vi "bundleArregloValores.vi"(8 "error in (no error)":errorcluster, 11 "ValoresControles":string[](array[string])=["marca 1", "modelo 1", "1231321", "", "", "Clase 1", "marca 1", "marca 1", "632131", "marca 1", "modelo 1", "654546"]) -> (0 "error out":errorcluster, 3 "output cluster":T1)   [LabVIEW 2019, in "Sonometro.lvclass"]
uses:
  Sonometro.lvclass
  Base de Datos/BD/Controles/cluster_equipos.ctl
  nombreControlesEquipo.ctl
  Base de Datos/Base de Datos.lvclass
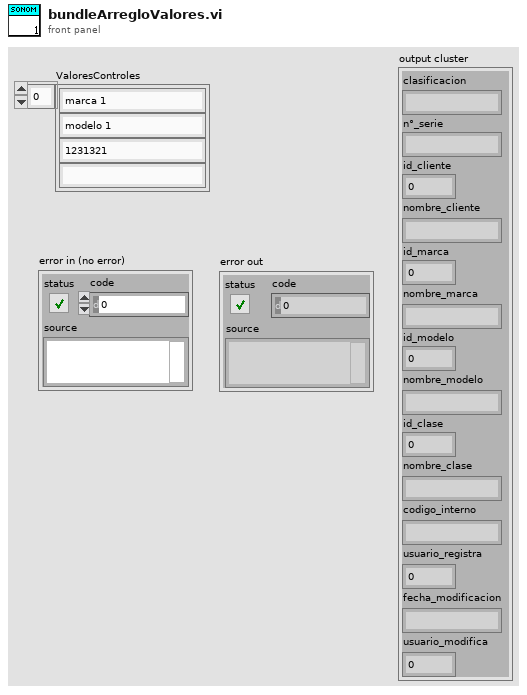
[diagram p1: front panel]
types:
  T1 = typedef "Base de Datos.lvclass/cluster_equipos.ctl" = cluster{"clasificacion":string, "n°_serie":string, "id_cliente":i32, "nombre_cliente":string, "id_marca":i32, "nombre_marca":string, "id_modelo":i32, "nombre_modelo":string, "id_clase":i32, "nombre_clase":string, "codigo_interno":string, "usuario_registra":i32, "fecha_modificacion":string, "usuario_modifica":i32}
  T2 = typedef "Sonometro.lvclass/nombreControlesEquipo.ctl" = string[]
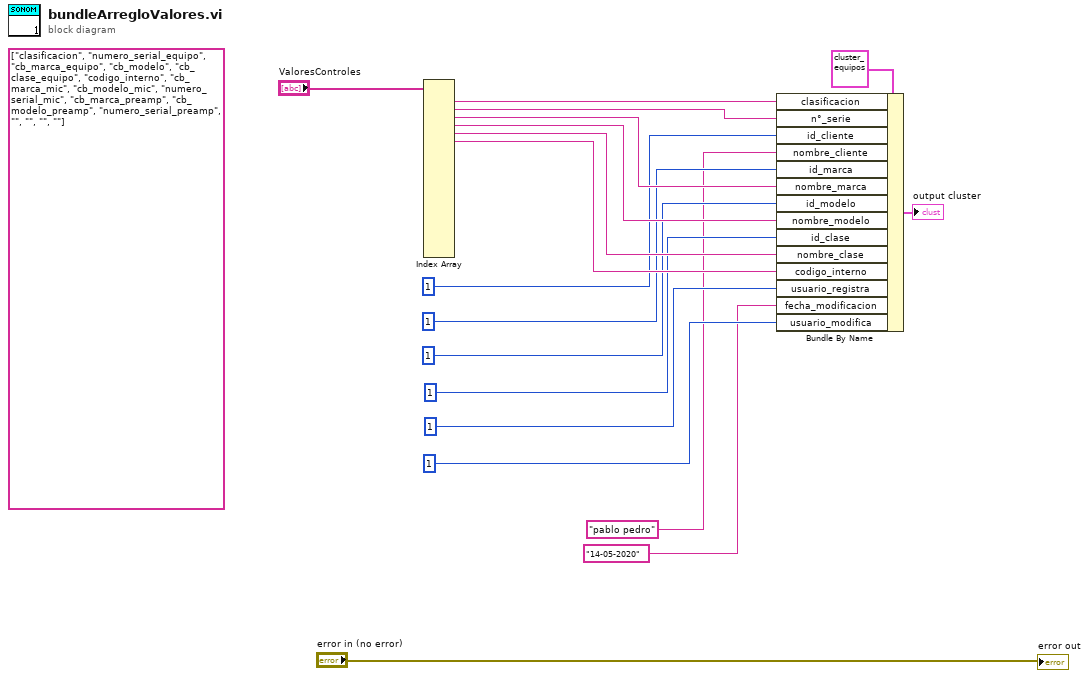
[diagram p0: block diagram]
diagram:
  (unwired) T2 ["clasificacion", "numero_serial_equipo", "cb_marca_equipo", "cb_modelo", "cb_clase_equipo", "codigo_interno", "cb_marca_mic", "cb_modelo_mic", "numero_serial_mic", "cb_marca_preamp", "cb_modelo_preamp", "numero_serial_preamp", "", "", "", ""] ("nombre_controles_equipo")
  n1 = Index Array(array="ValoresControles") -> (element #1=w16:string, element #2=w15:string, element #3=w14:string, element #4=w13:string, element #5=w12:string, element #6=w11:string)  [unwired: 20 in, 14 out]
  n2 = Bundle By Name(cluster=T1 {"clasificacion"="", "n°_serie"="", "id_cliente"=0, "nombre_cliente"="", "id_marca"=0, "nombre_marca"="", "id_modelo"=0, "nombre_modelo"="", "id_clase"=0, "nombre_clase"="", "codigo_interno"="", "usuario_registra"=0, "fecha_modificacion"="", "usuario_modifica"=0} ("cluster_equipos"), "clasificacion"=w16, "n°_serie"=w15, "id_cliente"=1, "nombre_cliente"="pablo pedro", "id_marca"=1 ("id_cliente"), "nombre_marca"=w14, "id_modelo"=1 ("id_cliente"), "nombre_modelo"=w13, "id_clase"=1 ("id_cliente"), "nombre_clase"=w12, "codigo_interno"=w11, "usuario_registra"=1 ("id_cliente"), "fecha_modificacion"="14-05-2020", "usuario_modifica"=1 ("id_cliente")) -> (→"output cluster":T1)
  "error out" <- "error in (no error)"
